vi "Func-엑셀 데이터를 그래프로 출력.vi"() -> ()   [LabVIEW 2015] (continued)
25\t-38.4\t-30.037\n25\t-38.24\t-30.037\n25\t-38.09\t-30.039\n25\t-37.93\t-30.042\n25\t-37.77\t-30.042\n25\t-37.59\t-30.043\n25\t-37.41\t-30.045\n25\t-37.23\t-30.045\n25\t-37.04\t-30.041\n25\t-36.85\t-30.041\n25\t-36.65\t-30.036\n25\t-36.44\t-30.038\n25\t-36.24\t-30.038\n25\t-36.03\t-30.038\n25\t-35.82\t-30.038\n25\t-35.61\t-30.036\n25\t-35.38\t-30.038\n25\t-35.15\t-30.046\n25\t-34.93\t-30.046\n25\t-34.7\t-30.048\n25\t-34.47\t-30.044\n25\t-34.24\t-30.043\n25\t-33.99\t-30.039\n25\t-33.75\t-30.036\n25\t-33.5\t-30.032\n25\t-33.25\t-30.032\n25\t-33.01\t-30.034\n25\t-32.75\t-30.036\n25\t-32.5\t-30.032\n25\t-32.24\t-30.026\n25\t-31.97\t-30.025\n25\t-31.7\t-30.027\n25\t-31.43\t-30.024\n25\t-31.16\t-30.021\n25\t-30.89\t-30.014\n25\t-30.61\t-30.014\n25\t-30.33\t-30.019\n25\t-30.04\t-30.02\n25\t-29.76\t-30.021\n25\t-29.48\t-30.016\n25\t-29.19\t-30.013\n25\t-28.89\t-30.01\n25\t-28.6\t-30.01\n25\t-28.31\t-30.009\n25\t-28.01\t-30.011\n25\t-27.71\t-30.004\n25\t-27.41\t-30.005\n25\t-27.1\t-29.999\n25\t-26.8\t-29.994\n25\t-26.49\t-29.989\n25\t-26.18\t-29.988\n25\t-25.87\t-29.988\n25\t-25.56\t-29.985\n25\t-25.25\t-29.977\n25\t-24.94\t-29.975\n25\t-24.62\t-29.974\n25\t-24.3\t-29.972\n25\t-23.98\t-29.966\n25\t-23.66\t-29.962\n25\t-23.34\t-29.954\n25\t-23.01\t-29.945\n25\t-22.68\t-29.941\n25\t-22.36\t-29.934\n25\t-22.04\t-29.932\n25\t-21.71\t-29.929\n25\t-21.38\t-29.927\n25\t-21.05\t-29.925\n25\t-20.72\t-29.919\n25\t-20.38\t-29.914\n25\t-20.04\t-29.904\n25\t-19.7\t-29.901\n25\t-19.38\t-29.889\n25\t-19.05\t-29.882\n25\t-18.71\t-29.877\n25\t-18.37\t-29.876\n25\t-18.03\t-29.866\n25\t-17.69\t-29.857\n25\t-17.34\t-29.848\n25\t-17\t-29.841\n25\t-16.67\t-29.834\n25\t-16.33\t-29.822\n25\t-15.98\t-29.817\n25\t-15.64\t-29.801\n25\t-15.3\t-29.791\n25\t-14.94\t-29.784\n25\t-14.6\t-29.775\n25\t-14.24\t-29.769\n25\t-13.89\t-29.755\n25\t-13.55\t-29.745\n25\t-13.2\t-29.732\n25\t-12.84\t-29.721\n25\t-12.32\t-29.7\n25\t-12.14\t-29.694\n25\t-11.79\t-29.688\n25\t-11.42\t-29.675\n25\t-11.06\t-29.664\n25\t-10.7\t-29.649\n25\t-10.33\t-29.632\n25\t-9.97\t-29.618\n25\t-9.61\t-29.602\n25\t-9.26\t-29.589\n25\t-8.89\t-29.573\n25\t-8.53\t-29.559\n25\t-8.17\t-29.539\n25\t-7.81\t-29.525\n25\t-7.45\t-29.513\n25\t-7.09\t-29.501\n25\t-6.75\t-29.482\n25\t-6.39\t-29.455\n25\t-6.03\t-29.432\n25\t-5.68\t-29.418\n25\t-5.32\t-29.402\n25\t-4.96\t-29.381\n25\t-4.61\t-29.364\n25\t-4.25\t-29.347\n25\t-3.89\t-29.329\n25\t-3.54\t-29.312\n25\t-3.18\t-29.289\n25\t-2.83\t-29.265\n25\t-2.47\t-29.241\n25\t-2.1\t-29.217\n25\t-1.74\t-29.195\n25\t-1.39\t-29.176\n25\t-1.04\t-29.147\n25\t-0.68\t-29.116\n25\t-0.33\t-29.091\n25\t0.01\t-29.071\n25\t0.36\t-29.048\n25\t0.71\t-29.03\n25\t1.06\t-29.002\n25\t1.4\t-28.975\n25\t1.75\t-28.949\n25\t2.1\t-28.917\n25\t2.45\t-28.89\n25\t2.8\t-28.867\n25\t3.15\t-28.84\n25\t3.5\t-28.813\n25\t3.85\t-28.786\n25\t4.2\t-28.758\n25\t4.54\t-28.733\n25\t4.88\t-28.701\n25\t5.22\t-28.671\n25\t5.57\t-28.645\n25\t5.92\t-28.611\n25\t6.27\t-28.58\n25\t6.62\t-28.553\n25\t6.96\t-28.519\n25\t7.3\t-28.483\n25\t7.65\t-28.449\n25\t8\t-28.415\n25\t8.36\t-28.377\n25\t8.71\t-28.344\n25\t9.06\t-28.308\n25\t9.42\t-28.273\n25\t9.77\t-28.246\n25\t10.11\t-28.205\n25\t10.45\t-28.17\n25\t10.78\t-28.127\n25\t11.12\t-28.089\n25\t11.45\t-28.057\n25\t11.8\t-28.016\n25\t12.13\t-27.973\n25\t12.47\t-27.937\n25\t12.81\t-27.895\n25\t13.14\t-27.847\n25\t13.47\t-27.802\n25\t13.81\t-27.762\n25\t14.13\t-27.721\n25\t14.45\t-27.683\n25\t14.76\t-27.635\n25\t15.08\t-27.589\n25\t15.39\t-27.54\n25\t15.7\t-27.5\n25\t16.01\t-27.454\n25\t16.31\t-27.409\n25\t16.6\t-27.365\n25\t16.9\t-27.313\n25\t17.19\t-27.267\n25\t17.47\t-27.217\n25\t17.75\t-27.166\n25\t18.01\t-27.124\n25\t18.26\t-27.072\n25\t18.63\t-26.991\n25\t18.76\t-26.966\n25\t19\t-26.907\n25\t19.22\t-26.854\n25\t19.45\t-26.805\n25\t19.65\t-26.753\n25\t19.85\t-26.696\n25\t20.04\t-26.647\n25\t20.23\t-26.588\n25\t20.41\t-26.522\n25\t20.57\t-26.461\n25\t20.73\t-26.409\n25\t20.88\t-26.35\n25\t21.02\t-26.295\n25\t21.15\t-26.232\n25\t21.28\t-26.175\n25\t21.41\t-26.124\n25\t21.51\t-26.06\n25\t21.68\t-25.967\n25\t21.72\t-25.939\n25\t21.82\t-25.872\n25\t21.9\t-25.806\n25\t21.97\t-25.748\n25\t22.04\t-25.686\n25\t22.11\t-25.618\n25\t22.17\t-25.554\n25\t22.22\t-25.482\n25\t22.27\t-25.409\n25\t22.3\t-25.353\n25\t22.34\t-25.282\n25\t22.37\t-25.219\n25\t22.39\t-25.153\n25\t22.4\t-25.093\n25\t22.42\t-25.013\n25\t22.43\t-24.936\n25\t22.43\t-24.872\n25\t22.44\t-24.76\n25\t22.44\t-24.731\n25\t22.43\t-24.664\n25\t22.41\t-24.589\n25\t22.4\t-24.508\n25\t22.39\t-24.444\n25\t22.38\t-24.368\n25\t22.36\t-24.288\n25\t22.33\t-24.217\n25\t22.31\t-24.14\n25\t22.29\t-24.066\n25\t22.26\t-23.999\n25\t22.22\t-23.913\n25\t22.19\t-23.83\n25\t22.15\t-23.758\n25\t22.11\t-23.681\n25\t22.07\t-23.596\n25\t22.03\t-23.527\n25\t21.95\t-23.4\n25\t21.93\t-23.365\n25\t21.88\t-23.293\n25\t21.83\t-23.208\n25\t21.77\t-23.122\n25\t21.73\t-23.041\n25\t21.68\t-22.965\n25\t21.62\t-22.887\n25\t21.57\t-22.796\n25\t21.52\t-22.723\n25\t21.48\t-22.632\n25\t21.43\t-22.545\n25\t21.4\t-22.472\n25\t21.35\t-22.388\n25\t21.32\t-22.299\n25\t21.28\t-22.219\n25\t21.24\t-22.126\n25\t21.22\t-22.038\n25\t21.17\t-21.915\n25\t21.15\t-21.877\n25\t21.13\t-21.786\n25\t21.1\t-21.704\n25\t21.08\t-21.613\n25\t21.06\t-21.521\n25\t21.04\t-21.444\n25\t21.02\t-21.358\n25\t21.01\t-21.268\n25\t21\t-21.189\n25\t20.99\t-21.088\n25\t20.98\t-20.996\n25\t20.97\t-20.918\n25\t20.97\t-20.834\n25\t20.97\t-20.738\n25\t20.97\t-20.657\n25\t20.97\t-20.554\n25\t20.97\t-20.422\n25\t20.97\t-20.382\n25\t20.97\t-20.289\n25\t20.97\t-20.191\n25\t20.97\t-20.112\n25\t20.98\t-20.021\n25\t20.99\t-19.926\n25\t21\t-19.842\n25\t21.02\t-19.741\n25\t21.04\t-19.644\n25\t21.06\t-19.562\n25\t21.07\t-19.471\n25\t21.09\t-19.375\n25\t21.12\t-19.294\n25\t21.14\t-19.196\n25\t21.15\t-19.105\n25\t21.18\t-19.023\n25\t21.2\t-18.925\n25\t21.23\t-18.828\n25\t21.25\t-18.745\n25\t21.28\t-18.649\n25\t21.31\t-18.55\n25\t21.33\t-18.463\n25\t21.37\t-18.368\n25\t21.4\t-18.27\n25\t21.42\t-18.191\n25\t21.45\t-18.093\n25\t21.48\t-17.997\n25\t21.5\t-17.898\n25\t21.53\t-17.814\n25\t21.56\t-17.716\n25\t21.59\t-17.617\n25\t21.62\t-17.532\n25\t21.65\t-17.436\n25\t21.68\t-17.342\n25\t21.7\t-17.257\n25\t21.73\t-17.154\n25\t21.77\t-17.014\n25\t21.78\t-16.97\n25\t21.81\t-16.874\n25\t21.85\t-16.77\n25\t21.87\t-16.689\n25\t21.9\t-16.587\n25\t21.93\t-16.494\n25\t21.96\t-16.409\n25\t21.99\t-16.313\n25\t22.03\t-16.212\n25\t22.06\t-16.113\n25\t22.09\t-16.028\n25\t22.12\t-15.929\n25\t22.15\t-15.836\n25\t22.19\t-15.751\n25\t22.21\t-15.655\n25\t22.25\t-15.546\n25\t22.28\t-15.464\n25\t22.31\t-15.362\n25\t22.35\t-15.224\n25\t22.38\t-15.13\n25\t22.39\t-15.086\n25\t22.42\t-14.987\n25\t22.45\t-14.906\n25\t22.48\t-14.809\n25\t22.51\t-14.723\n25\t22.54\t-14.636\n25\t22.57\t-14.535\n25\t22.59\t-14.429\n25\t22.62\t-14.343\n25\t22.66\t-14.249\n25\t22.67\t-14.148\n25\t22.7\t-14.052\n25\t22.74\t-13.971\n25\t22.76\t-13.877\n25\t22.78\t-13.784\n25\t22.81\t-13.692\n25\t22.85\t-13.531\n25\t22.86\t-13.489\n25\t22.89\t-13.409\n25\t22.92\t-13.313\n25\t22.95\t-13.218\n25\t22.98\t-13.13\n25\t23.01\t-13.032\n25\t23.03\t-12.937\n25\t23.06\t-12.857\n25\t23.09\t-12.76\n25\t23.11\t-12.659\n25\t23.14\t-12.579\n25\t23.16\t-12.481\n25\t23.19\t-12.389\n25\t23.21\t-12.304\n25\t23.24\t-12.211\n25\t23.26\t-12.111\n25\t23.28\t-12.029\n25\t23.3\t-11.927\n25\t23.35\t-11.788\n25\t23.36\t-11.747\n25\t23.37\t-11.652\n25\t23.4\t-11.56\n25\t23.42\t-11.479\n25\t23.44\t-11.382\n25\t23.46\t-11.285\n25\t23.48\t-11.207\n25\t23.5\t-11.113\n25\t23.53\t-11.019\n25\t23.55\t-10.932\n25\t23.56\t-10.837\n25\t23.59\t-10.742\n25\t23.61\t-10.648\n25\t23.63\t-10.568\n25\t23.64\t-10.475\n25\t23.66\t-10.385\n25\t23.68\t-10.305\n25\t23.71\t-10.214\n25\t23.73\t-10.115\n25\t23.75\t-10.033\n25\t23.77\t-9.932\n25\t23.79\t-9.842\n25\t23.81\t-9.766\n25\t23.82\t-9.675\n25\t23.84\t-9.584\n25\t23.87\t-9.5\n25\t23.89\t-9.411\n25\t23.9\t-9.315\n25\t23.93\t-9.236\n25\t23.95\t-9.143\n25\t23.97\t-9.049\n25\t23.99\t-8.969\n25\t24\t-8.877\n25\t24.02\t-8.792\n25\t24.05\t-8.663\n25\t24.05\t-8.623\n25\t24.08\t-8.525\n25\t24.08\t-8.448\n25\t24.1\t-8.363\n25\t24.12\t-8.273\n25\t24.14\t-8.175\n25\t24.16\t-8.094\n25\t24.17\t-8.007\n25\t24.18\t-7.924\n25\t24.2\t-7.85\n25\t24.22\t-7.765\n25\t24.23\t-7.673\n25\t24.25\t-7.597\n25\t24.26\t-7.5\n25\t24.27\t-7.414\n25\t24.28\t-7.341\n25\t24.3\t-7.252\n25\t24.32\t-7.158\n25\t24.34\t-7.032\n25\t24.35\t-6.949\n25\t24.35\t-6.91\n25\t24.37\t-6.831\n25\t24.38\t-6.746\n25\t24.4\t-6.657\n25\t24.41\t-6.584\n25\t24.42\t-6.496\n25\t24.44\t-6.411\n25\t24.44\t-6.34\n25\t24.46\t-6.253\n25\t24.48\t-6.167\n25\t24.49\t-6.097\n25\t24.5\t-6.011\n25\t24.51\t-5.926\n25\t24.53\t-5.848\n25\t24.53\t-5.762\n25\t24.55\t-5.674\n25\t24.56\t-5.601\n25\t24.58\t-5.518\n25\t24.59\t-5.43\n25\t24.6\t-5.358\n25\t24.62\t-5.27\n25\t24.62\t-5.191\n25\t24.63\t-5.119\n25\t24.64\t-5.037\n25\t24.65\t-4.957\n25\t24.66\t-4.889\n25\t24.67\t-4.807\n25\t24.68\t-4.721\n25\t24.69\t-4.63\n25\t24.7\t-4.557\n25\t24.71\t-4.471\n25\t24.71\t-4.391\n25\t24.72\t-4.322\n25\t24.73\t-4.242\n25\t24.74\t-4.173\n25\t24.75\t-4.052\n25\t24.75\t-4.021\n25\t24.76\t-3.954\n25\t24.77\t-3.875\n25\t24.78\t-3.791\n25\t24.79\t-3.704\n25\t24.8\t-3.631\n25\t24.8\t-3.549\n25\t24.8\t-3.471\n25\t24.81\t-3.402\n25\t24.81\t-3.322\n25\t24.82\t-3.241\n25\t24.82\t-3.168\n25\t24.83\t-3.09\n25\t24.83\t-3.009\n25\t24.84\t-2.945\n25\t24.84\t-2.868\n25\t24.85\t-2.759\n25\t24.86\t-2.726\n25\t24.87\t-2.644\n25\t24.87\t-2.563\n25\t24.88\t-2.498\n25\t24.88\t-2.423\n25\t24.89\t-2.35\n25\t24.89\t-2.282\n25\t24.89\t-2.204\n25\t24.89\t-2.125\n25\t24.9\t-2.062\n25\t24.91\t-1.966\n25\t24.91\t-1.954\n25\t24.91\t-1.931\n25\t24.91\t-1.911\n25\t24.91\t-1.902\n25\t24.91\t-1.876\n25\t24.92\t-1.855\n25\t24.92\t-1.843\n25\t24.92\t-1.822\n25\t24.92\t-1.8\n25\t24.92\t-1.789\n25\t24.92\t-1.766\n25\t24.93\t-1.745\n25\t24.93\t-1.735\n25\t24.93\t-1.712\n25\t24.93\t-1.688\n25\t24.92\t-1.676\n25\t24.92\t-1.658\n25\t24.93\t-1.635\n25\t24.93\t-1.624\n25\t24.93\t-1.6\n25\t24.93\t-1.579\n25\t24.93\t-1.566\n25\t24.93\t-1.546\n25\t24.94\t-1.524\n25\t24.94\t-1.509\n25\t24.94\t-1.487\n25\t24.94\t-1.469\n25\t24.94\t-1.459\n25\t24.94\t-1.437\n25\t24.95\t-1.415\n25\t24.95\t-1.405\n25\t24.95\t-1.385\n25\t24.95\t-1.365\n25\t24.95\t-1.354\n25\t24.95\t-1.333\n25\t24.96\t-1.311\n25\t24.96\t-1.303\n25\t24.96\t-1.284\n25\t24.96\t-1.262\n25\t24.96\t-1.251\n25\t24.96\t-1.228\n25\t24.96\t-1.206\n25\t24.96\t-1.195\n25\t24.97\t-1.175\n25\t24.97\t-1.151\n25\t24.97\t-1.142\n25\t24.97\t-1.121\n25\t24.97\t-1.099\n25\t24.97\t-1.087\n25\t24.97\t-1.062\n25\t24.97\t-1.041\n25\t24.97\t-1.03\n25\t24.97\t-1.007\n25\t24.97\t-0.987\n25\t24.97\t-0.963\n25\t24.97\t-0.95\n25\t24.97\t-0.932\n25\t24.98\t-0.922\n25\t24.98\t-0.899\n25\t24.98\t-0.879\n25\t24.98\t-0.86\n25\t24.98\t-0.85\n25\t24.98\t-0.828\n25\t24.98\t-0.808\n25\t24.98\t-0.799\n25\t24.98\t-0.776\n25\t24.98\t-0.759\n25\t24.98\t-0.748\n25\t24.98\t-0.725\n25\t24.98\t-0.716\n25\t24.98\t-0.696\n25\t24.98\t-0.676\n25\t24.98\t-0.652\n25\t24.98\t-0.643\n25\t24.98\t-0.623\n25\t24.98\t-0.603\n25\t24.98\t-0.591\n25\t24.99\t-0.571\n25\t24.99\t-0.546\n25\t24.99\t-0.536\n25\t24.99\t-0.514\n25\t24.99\t-0.489\n25\t24.99\t-0.478\n25\t25\t-0.456\n25\t25\t-0.438\n25\t25\t-0.428\n25\t25\t-0.407\n25\t25\t-0.385\n25\t25\t-0.374\n25\t25\t-0.354\n25\t25\t-0.334\n25\t25.01\t-0.325\n25\t25.01\t-0.305\n25\t25.01\t-0.285\n25\t25.01\t-0.274\n25\t25.01\t-0.254\n25\t25.01\t-0.229\n25\t25.01\t-0.217\n25\t25.01\t-0.199\n25\t25.01\t-0.179\n25\t25.01\t-0.168\n25\t25.01\t-0.149\n25\t25.01\t-0.128\n25\t25.02\t-0.116\n25\t25.02\t-0.096\n25\t25.02\t-0.077\n25\t25.02\t-0.068\n25\t25.02\t-0.049\n25\t25.02\t-0.03\n25\t25.02\t-0.021\n25\t25.02\t0.002\n25\t25.02\t0.022\n25\t25.02\t0.031\n25\t25.03\t0.055\n25\t25.03\t0.073\n25\t25.03\t0.084\n25\t25.03\t0.106\n25\t25.03\t0.126\n25\t25.03\t0.138\n25\t25.03\t0.159\n25\t25.03\t0.179\n25\t25.03\t0.188\n25\t25.03\t0.211\n25\t25.04\t0.23\n25\t25.04\t0.24\n25\t25.04\t0.26\n25\t25.04\t0.282\n25\t25.04\t0.29\n25\t25.04\t0.31\n25\t25.04\t0.33\n25\t25.04\t0.348\n25\t25.04\t0.361\n25\t25.04\t0.383\n25\t25.04\t0.393\n25\t25.04\t0.412\n25\t25.04\t0.434\n25\t25.04\t0.445\n25\t25.04\t0.464\n25\t25.04\t0.482\n25\t25.04\t0.502\n25\t25.04\t0.514\n25\t25.04\t0.533\n25\t25.04\t0.555\n25\t25.05\t0.564\n25\t25.05\t0.584\n25\t25.04\t0.607\n25\t25.04\t0.616\n25\t25.03\t0.635\n25\t25.03\t0.654\n25\t25.02\t0.667\n25\t25.02\t0.686\n25\t25.01\t0.705\n25\t25.01\t0.714\n25\t25\t0.735\n25\t25\t0.752\n25\t25.01\t0.764\n25\t25.01\t0.784\n25\t25.01\t0.802\n25\t25.01\t0.813\n25\t25.01\t0.834\n25\t25.01\t0.855\n25\t25.01\t0.864\n25\t25.01\t0.885\n25\t25.01\t0.907\n25\t25.01\t0.92\n25\t25.01\t0.94\n25\t25.01\t0.96\n25\t25.01\t0.968\n25\t25.01\t0.987\n25\t25.01\t1.007\n25\t25.01\t1.016\n25\t25.01\t1.036\n25\t25.01\t1.056\n25\t25.01\t1.064\n25\t25.01\t1.085\n25\t25.01\t1.105\n25\t25.01\t1.113\n25\t25.01\t1.134\n25\t25.01\t1.155\n25\t25.01\t1.167\n25\t25.01\t1.187\n25\t25.01\t1.206\n25\t25.01\t1.216\n25\t25.01\t1.237\n25\t25.01\t1.258\n25\t25.01\t1.27\n25\t25.01\t1.292\n25\t25.01\t1.311\n25\t25.01\t1.321\n25\t25.01\t1.34\n25\t25.01\t1.356\n25\t25.01\t1.366\n25\t25.01\t1.387\n25\t25.01\t1.405\n25\t25.01\t1.417\n25\t25.01\t1.437\n25\t25.01\t1.457\n25\t25.01\t1.466\n25\t25.01\t1.484\n25\t25.01\t1.502\n25\t25.01\t1.513\n25\t25.01\t1.532\n25\t25.01\t1.556\n25\t25.01\t1.566\n25\t25.01\t1.585\n25\t25.01\t1.605\n25\t25.01\t1.612\n25\t25.01\t1.629\n25\t25.01\t1.645\n25\t25.01\t1.656\n25\t25.01\t1.677\n25\t25.01\t1.696\n25\t25.01\t1.707\n25\t25.01\t1.725\n25\t25.01\t1.742\n25\t25.01\t1.751\n25\t25.01\t1.769\n25\t25.01\t1.79\n25\t25.01\t1.8\n25\t25.01\t1.819\n25\t25.01\t1.84\n25\t25.01\t1.848\n25\t25.01\t1.869\n25\t25.01\t1.888\n25\t25.01\t1.896\n25\t25.01\t1.918\n25\t25.01\t1.939\n25\t25.01\t1.948\n25\t25.01\t1.969\n25\t25.01\t1.987\n25\t25.01\t1.996\n25\t25.01\t2.019\n25\t25.01\t2.036\n25\t25.01\t2.054\n25\t25.01\t2.062\n25\t25.01\t2.082\n25\t25.01\t2.093\n25\t25.01\t2.111\n25\t25.01\t2.13\n25\t25.01\t2.15\n25\t25.01\t2.159\n25\t25.01\t2.178\n25\t25.01\t2.2\n25\t25.01\t2.207\n25\t25.01\t2.231\n25\t25.01\t2.241\n25\t25.01\t2.259\n25\t25.01\t2.278\n25\t25.01\t2.287\n25\t25.01\t2.307\n25\t25.01\t2.327\n25\t25.01\t2.336\n25\t25.01\t2.354\n25\t25.01\t2.373\n25\t25.01\t2.392\n25\t25.01\t2.403\n25\t25.01\t2.42\n25\t25.01\t2.431\n25\t25.01\t2.451\n25\t25.01\t2.47\n25\t25.01\t2.48\n25\t25.01\t2.5\n25\t25.01\t2.515\n25\t25.01\t2.536\n25\t25.01\t2.544\n25\t25.01\t2.562\n25\t25.01\t2.58\n25\t25.01\t2.589\n25\t25.01\t2.608\n25\t25.01\t2.616\n25\t25.01\t2.634\n25\t25.01\t2.656\n25\t25.01\t2.673\n25\t25.01\t2.682\n25\t25.01\t2.704\n25\t25.01\t2.722\n25\t25.01\t2.732\n25\t25.01\t2.75\n25\t25.01\t2.768\n25\t25.01\t2.78\n25\t25.01\t2.799\n25\t25.01\t2.816\n25\t25.01\t2.824\n25\t25.01\t2.839\n25\t25.01\t2.857\n25\t25.01\t2.866\n25\t25.01\t2.884\n25\t25.01\t2.904\n25\t25.01\t2.913\n25\t25.01\t2.934\n25\t25.01\t2.955\n25\t25.01\t2.963\n25\t25.01\t2.98\n25\t25.01\t3.002\n25\t25.01\t3.013\n25\t25.01\t3.034\n25\t25.01\t3.053\n25\t25.01\t3.064\n25\t25.01\t3.085\n25\t25.01\t3.104\n25\t25.01\t3.113\n25\t25.01\t3.13\n25\t25.01\t3.146\n25\t25.01\t3.157\n25\t25.01\t3.177\n25\t25.01\t3.195\n25\t25.01\t3.203\n25\t25.01\t3.221\n25\t25.01\t3.24\n25\t25.01\t3.248\n25\t25.01\t3.264\n25\t25.01\t3.282\n25\t25.01\t3.293\n25\t25.01\t3.311\n25\t25.01\t3.329\n25\t25.01\t3.338\n25\t25.01\t3.359\n25\t25.01\t3.379\n25\t25.01\t3.389\n25\t25.01\t3.411\n25\t25.01\t3.43\n25\t25.01\t3.44\n25\t25.01\t3.457\n25\t25.01\t3.479\n25\t25.01\t3.487\n25\t25.01\t3.509\n25\t25.01\t3.526\n25\t25.01\t3.535\n25\t25.01\t3.552\n25\t25.01\t3.57\n25\t25.01\t3.581\n25\t25.01\t3.596\n25\t25.01\t3.614\n25\t25.01\t3.622\n25\t25.01\t3.643\n25\t25.01\t3.659\n25\t25.01\t3.668\n25\t25.01\t3.684\n25\t25.01\t3.706\n25\t25.01\t3.716\n25\t25.01\t3.732\n25\t25.01\t3.749\n25\t25.01\t3.757\n25\t25.01\t3.777\n25\t25.01\t3.795\n25\t25.01\t3.805\n25\t25.01\t3.821\n25\t25.01\t3.841\n25\t25.01\t3.848\n25\t25.01\t3.866\n25\t25.01\t3.882\n25\t25.01\t3.892\n25\t25.01\t3.914\n25\t25.01\t3.931\n25\t25.01\t3.94\n25\t25.01\t3.958\n25\t25.01\t3.977\n25\t25.01\t3.986\n25\t25.01\t4.009\n25\t25.01\t4.026\n25\t25.01\t4.037\n25\t25.01\t4.057\n25\t25.01\t4.074\n25\t25.01\t4.083\n25\t25.01\t4.1\n25\t25.01\t4.118\n25\t25.01\t4.126\n25\t25.01\t4.146\n25\t25.01\t4.164\n25\t25.01\t4.182\n25\t25.01\t4.189\n25\t25.01\t4.209\n25\t25.01\t4.219\n25\t25.01\t4.234\n25\t25.01\t4.255\n25\t25.01\t4.265\n25\t25.01\t4.286\n25\t25.01\t4.306\n25\t25.01\t4.325\n25\t25.01\t4.333\n25\t25.01\t4.352\n25\t25.01\t4.37\n25\t25.01\t4.379\n25\t25.01\t4.398\n25\t25.01\t4.415\n25\t25.01\t4.427\n25\t25.01\t4.444\n25\t25.01\t4.462\n25\t25.01\t4.471\n25\t25.01\t4.491\n25\t25.01\t4.51\n25\t25.01\t4.519\n25\t25.01\t4.536\n25\t25.01\t4.555\n25\t25.01\t4.565\n25\t25.01\t4.584\n25\t25.01\t4.602\n25\t25.02\t4.611\n25\t25.02\t4.629\n25\t25.01\t4.648\n25\t25.01\t4.657\n25\t25.01\t4.672\n25\t25.01\t4.689\n25\t25.02\t4.698\n25\t25.02\t4.717\n25\t25.02\t4.736\n25\t25.02\t4.745\n25\t25.02\t4.764\n25\t25.02\t4.782\n25\t25.02\t4.791\n25\t25.02\t4.809\n25\t25.02\t4.827\n25\t25.02\t4.834\n25\t25.02\t4.854\n25\t25.02\t4.873\n25\t25.02\t4.884\n25\t25.02\t4.897\n25\t25.02\t4.917\n25\t25.02\t4.925\n25\t25.02\t4.942\n25\t25.02\t4.96\n25\t25.02\t4.97\n25\t25.02\t4.987\n25\t25.02\t5.005\n25\t25.02\t5.014\n25\t25.02\t5.032\n25\t25.02\t5.05\n25\t25.02\t5.059\n25\t25.02\t5.079\n25\t25.02\t5.093\n25\t25.02\t5.104\n25\t25.02\t5.12\n25\t25.02\t5.136\n25\t25.02\t5.144\n25\t25.02\t5.165\n25\t25.02\t5.18\n25\t25.02\t5.189\n25\t25.02\t5.206\n25\t25.02\t5.225\n25\t25.02\t5.234\n25\t25.02\t5.252\n25\t25.02\t5.274\n25\t25.02\t5.283\n25\t25.02\t5.302\n25\t25.02\t5.32\n25\t25.02\t5.33\n25\t25.02\t5.344\n25\t25.03\t5.365\n25\t25.03\t5.375\n25\t25.03\t5.393\n25\t25.03\t5.411\n25\t25.03\t5.419\n25\t25.03\t5.439\n25\t25.03\t5.455\n25\t25.03\t5.464\n25\t25.03\t5.479\n25\t25.03\t5.497\n25\t25.03\t5.505\n25\t25.03\t5.522\n25\t25.03\t5.539\n25\t25.03\t5.548\n25\t25.03\t5.568\n25\t25.03\t5.585\n25\t25.03\t5.593\n25\t25.03\t5.608\n25\t25.03\t5.625\n25\t25.03\t5.635\n25\t25.03\t5.655\n25\t25.03\t5.674\n25\t25.03\t5.693\n25\t25.03\t5.703\n25\t25.03\t5.72\n25\t25.03\t5.738\n25\t25.03\t5.747\n25\t25.03\t5.766\n25\t25.03\t5.786\n25\t25.03\t5.794\n25\t25.03\t5.811\n25\t25.03\t5.827\n25\t25.03\t5.837\n25\t25.03\t5.857\n25\t25.03\t5.873\n25\t25.03\t5.882\n25\t25.03\t5.902\n25\t25.03\t5.918\n25\t25.03\t5.927\n25\t25.03\t5.943\n25\t25.03\t5.957\n25\t25.03\t5.966\n25\t25.03\t5.986\n25\t25.03\t6.004\n25\t25.03\t6.013\n25\t25.03\t6.031\n25\t25.03\t6.05\n25\t25.03\t6.059\n25\t25.03\t6.075\n25\t25.03\t6.093\n25\t25.03\t6.102\n25\t25.03\t6.12\n25\t25.03\t6.141\n25\t25.03\t6.148\n25\t25.03\t6.163\n25\t25.03\t6.181\n25\t25.03\t6.189\n25\t25.03\t6.202\n25\t25.03\t6.221\n25\t25.03\t6.229\n25\t25.03\t6.248\n25\t25.03\t6.262\n25\t25.03\t6.27\n25\t25.03\t6.29\n25\t25.03\t6.306\n25\t25.03\t6.316\n25\t25.03\t6.336\n25\t25.03\t6.356\n25\t25.03\t6.363\n25\t25.03\t6.382\n25\t25.02\t6.4\n25\t25.02\t6.411\n25\t25.02\t6.429\n25\t25.02\t6.449\n25\t25.03\t6.458\n25\t25.03\t6.473\n25\t25.03\t6.491\n25\t25.03\t6.5\n25\t25.03\t6.517\n25\t25.03\t6.531\n25\t25.03\t6.541\n25\t25.03\t6.561\n25\t25.02\t6.577\n25\t25.02\t6.584\n25\t25.02\t6.601\n25\t25.02\t6.617\n25\t25.02\t6.629\n25\t25.02\t6.645\n25\t25.02\t6.661\n25\t25.02\t6.668\n25\t25.03\t6.685\n25\t25.03\t6.705\n25\t25.03\t6.711\n25\t25.03\t6.725\n25\t25.03\t6.743\n25\t25.03\t6.752\n25\t25.03\t6.768\n25\t25.03\t6.786\n25\t25.03\t6.792\n25\t25.03\t6.81\n25\t25.03\t6.828\n25\t25.03\t6.838\n25\t25.02\t6.857\n25\t25.02\t6.872\n25\t25.02\t6.882\n25\t25.02\t6.9\n25\t25.02\t6.916\n25\t25.02\t6.923\n25\t25.02\t6.94\n25\t25.02\t6.957\n25\t25.02\t6.977\n25\t25.02\t6.983\n25\t25.02\t6.999\n25\t25.02\t7.016\n25\t25.02\t7.024\n25\t25.02\t7.041\n25\t25.02\t7.061\n25\t25.02\t7.07\n25\t25.02\t7.087\n25\t25.02\t7.107\n25\t25.02\t7.116\n25\t25.02\t7.134\n25\t25.02\t7.15\n25\t25.02\t7.161\n25\t25.02\t7.181\n25\t25.02\t7.197\n25\t25.02\t7.205\n25\t25.02\t7.223\n25\t25.02\t7.24\n25\t25.02\t7.25\n25\t25.02\t7.267\n25\t25.02\t7.282\n25\t25.02\t7.291\n25\t25.02\t7.307\n25\t25.02\t7.323\n25\t25.02\t7.332\n25\t25.02\t7.35\n25\t25.02\t7.369\n25\t25.02\t7.377\n25\t25.02\t7.393\n25\t25.02\t7.41\n25\t25.02\t7.418\n25\t25.02\t7.437\n25\t25.02\t7.454\n25\t25.02\t7.463\n25\t25.02\t7.479\n25\t25.02\t7.498\n25\t25.02\t7.506\n25\t25.02\t7.521\n25\t25.02\t7.539\n25\t25.02\t7.546\n25\t25.02\t7.58\n"
  out "Graph 2":cluster{dbl[], dbl[]}[](graph)
  out "Graph 1":cluster{dbl[], dbl[]}[](graph)=[{array[36549 elements], [0.0003128, 0.00400914, 0.04822016, 0.09243478, 0.13661741, 0.18088003, 0.22513907, 0.26934129, 0.31354249, 0.35775453, 0.40194234, 0.44613013, 0.49034372, 0.53449279, 0.57871258, 0.62287194, 0.6670804, 0.71124184, 0.755328, 0.79956377, 0.84357244, 0.88760281, 0.93174618, 0.97576469, 1.01980484, 1.06384337, 1.10792947, 1.15197122, 1.19586015, 1.23986363, 1.28386247, 1.28381348, 1.24059355, 1.19588339, 1.15184271, 1.10791147, 1.06387436, 1.0198667, 0.97577345, 0.93180454, 0.88765496, 0.84360033, 0.79950494, 0.75538582, 0.71119487, 0.6671325, 0.62288386, 0.57876468, 0.53458673, 0.49045056, 0.44623077, 0.40202236, 0.35782215, 0.31363541, 0.26943782, 0.22521442, 0.18101114, 0.13677071, 0.09252615, 0.048247, 0.00409276, 0.00031384]}]
